vi "Unit test-POI group interface.vi"() -> ()   [LabVIEW 2020]
panel:
  in  "New group (F)":bool
  in  "Do it":bool
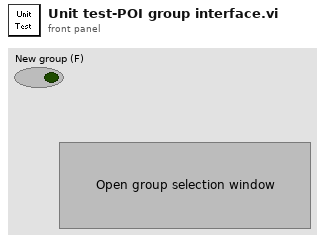
[diagram p1: front panel]
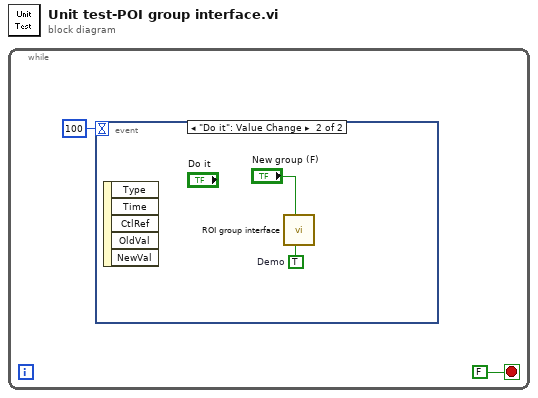
[diagram p0: block diagram]
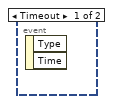
[diagram p2: hidden frame]
diagram:
  n1 = while {
    stop <- FALSE stop-if-true
    n2 = event shown="[1] \"Do it\": Value Change" {
      selector: _ -> [_ _]
      dyn-events: _ -> [_ _]
      timeout: 100 -> [_ _]
      event Timeout {
        n3 = event-data() -> ()  [unwired: 1 in, 2 out]
      }
      event "Do it": Value Change {
        w4 = TRUE  # Demo
        n4 = event-data() -> ()  [unwired: 1 in, 5 out]
        n5 = call "ROI group interface.vi"("Demo (F)"=w4, "New group (F)"="New group (F)") -> ()  [unwired: 7 in, 3 out]
      }
    }
  }
